vi "TRF to TSP Plot_09_21_12a_JW.vi"(8 "Transport Graph Properties":T1={"Transport Line Size"=0, "Transport Line Color"=16774656} {"Transport Line Size" items=["Extra Small", "Small", "Medium", "Large", "Extra Large"]}, 9 "No Transport File":path=path "\\\\acad1\\physics/Jurchescu-group/JW-PD/Mega Awesome/No Transport File.txt", 10 "Transport Folder":path, 11 "Transfer File":path) -> (1 "Transport":cluster{ext[], ext[]}[](graph), 2 "Transport File":path, 3 "Transport Name":string)   [LabVIEW 2012]
uses:
  <vilib>/Utility/file.llb/Read From Spreadsheet File (string).vi
  <vilib>/regexp/Match Regular Expression.xnode
panel:
  in  "default (0 dbl)":ext format="%.2e"
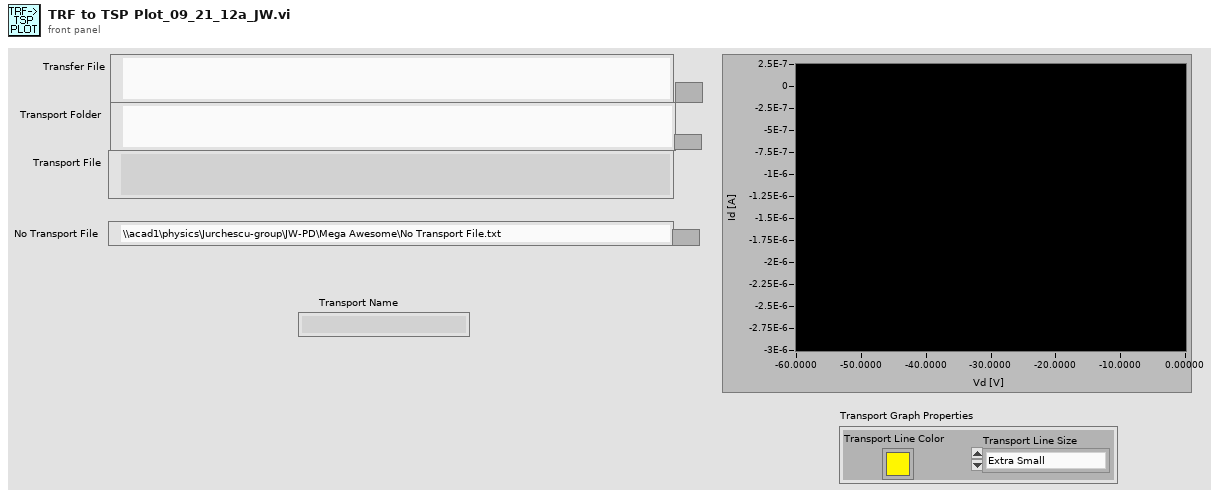
[diagram p1: front panel]
types:
  T1 = cluster{"Transport Line Size":u16, "Transport Line Color":u32}
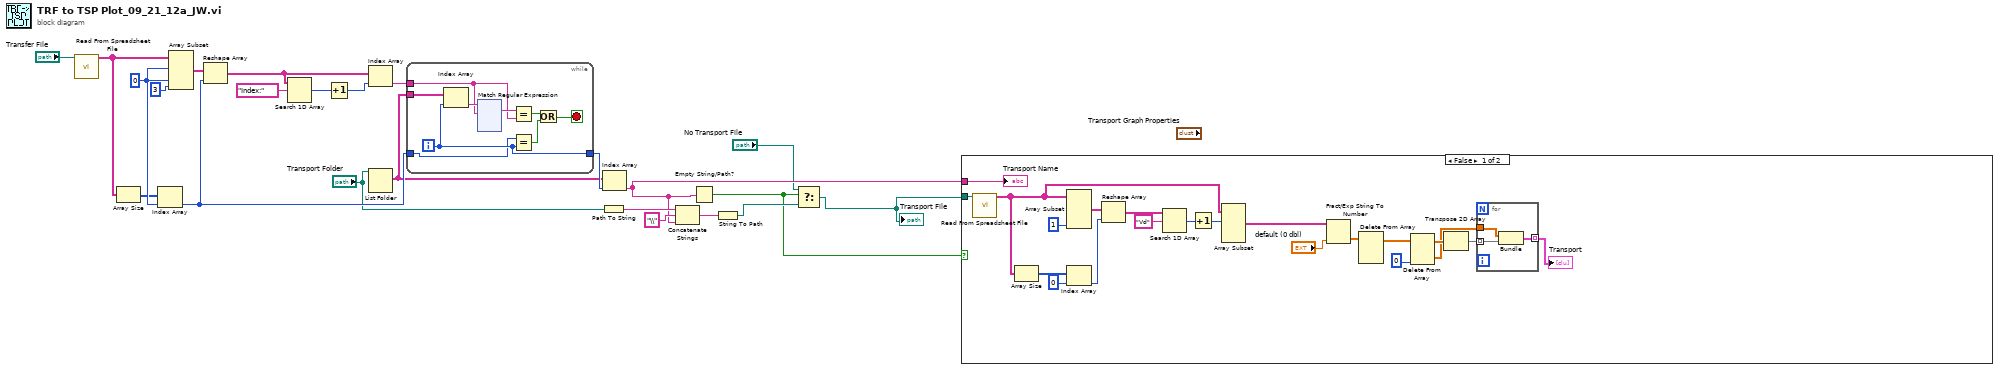
[diagram p0: block diagram]
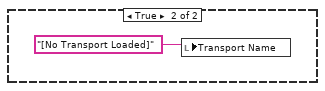
[diagram p2: hidden frame]
diagram:
  w22 = 0
  n1 = call-poly <vilib>:"Read From Spreadsheet File.vi"("file path (dialog if empty)"="Transfer File") -> ("all rows"=w18:string[][])  [unwired: 6 in, 4 out]
  n2 = Array Size(array=w18) -> (size(s)=w21:i32[])
  n3 = Index Array(array=w21, index=w22) -> (element=w12:i32)
  n4 = Array Subset(array=w18, index (row)=w22, index (col)=w22, length (col)=3) -> (w20:string[][])  [unwired: 1 in]
  n5 = Reshape Array(w20, w12) -> (w15:string[])
  n6 = Search 1D Array(1D array=w15, element="Index:") -> (index of element=w17:i32)  [unwired: 1 in]
  n7 = Increment(x=w17) -> (x+1=w14:i32)
  n8 = Index Array(array=w15, index=w14) -> (element=w13:string)
  n9 = List Folder(path="Transport Folder") -> (filenames=w9:string[])  [unwired: 3 in, 3 out]
  n10 = while {
    tunnel: w9 -> [w31]
    tunnel: w13 -> [w29]
    tunnel: [w28] -> w10
    tunnel: w12 -> [w27]
    i -> [w28]
    stop <- w24 stop-if-true
    n11 = Index Array(array=w31, index=w28) -> (element=w32:string)
    n12 = xnode "Match Regular Expression"("input string"=w32, "regular expression"=w29) -> ("whole match"=w30:string)  [unwired: 4 in, 4 out]
    n13 = Equal?(x=w30, y=w29) -> (x = y?=w26:bool)
    n14 = Equal?(x=w27, y=w28) -> (x = y?=w25:bool)
    n15 = Or(x=w26, y=w25) -> (x .or. y?=w24:bool)
  }
  n16 = Path To String(path="Transport Folder") -> (string=w6:string)
  n17 = Index Array(array=w9, index=w10) -> (element=w3:string)
  n18 = Concatenate Strings(w6, "\\", w3) -> (w7:string)
  n19 = Empty String/Path?(string/path=w3) -> (empty?=w1:bool)
  n20 = String To Path(string=w7) -> (path=w4:path)
  n21 = Select(t="No Transport File", s=w1, f=w4) -> (s? t:f=w5:path)
  "Transport File" <- w5
  n22 = case shown="False" w1 {
    tunnel: w5 -> [w164 _]
    tunnel: w3 -> [w144 _]
    frame False {
      n23 = call-poly <vilib>:"Read From Spreadsheet File.vi"("file path (dialog if empty)"=w164) -> ("all rows"=w157:string[][])  [unwired: 6 in, 4 out]
      n24 = Array Size(array=w157) -> (size(s)=w163:i32[])
      n25 = Array Subset(array=w157, length (col)=1) -> (w159:string[][])  [unwired: 3 in]
      n26 = Index Array(array=w163, index=0) -> (element=w152:i32)
      n27 = Reshape Array(w159, w152) -> (w158:string[])
      n28 = Search 1D Array(1D array=w158, element="Vd") -> (index of element=w156:i32)  [unwired: 1 in]
      n29 = Increment(x=w156) -> (x+1=w155:i32)
      n30 = Array Subset(array=w157, index (row)=w155) -> (w153:string[][])  [unwired: 3 in]
      n31 = Fract/Exp String To Number(string=w153, default (0 dbl)="default (0 dbl)") -> (number=w147:ext[][])  [unwired: 2 in, 1 out]
      n32 = Delete From Array(array=w147) -> (array with subset deleted=w146:ext[][])  [unwired: 3 in, 1 out]
      n33 = Delete From Array(array=w146, index (col)=0 ("Deaktivierter Index (Spalte)")) -> (deleted portion=w149:ext[], array with subset deleted=w150:ext[][])  [unwired: 2 in]
      n34 = Transpose 2D Array(2D array=w150) -> (transposed array=w151:ext[][])
      n35 = for {
        tunnel: w149 -> [w166]
        tunnel: w151 -> [w167] mode=indexing
        tunnel: [w165] -> w145 mode=indexing
        n36 = Bundle(w166, w167) -> (w165:cluster{ext[], ext[]})  [unwired: 1 in]
      }
      "Transport" <- w145
      "Transport Name" <- w144
    }
    frame True {
      n37 = local write "Transport Name"("[No Transport Loaded]") -> ()
    }
  }
